vi "TAT_Start.vi"(8 "error In":errorcluster) -> (0 "error out":errorcluster)   [LabVIEW 2017]
uses:
  <vilib>/Utility/error.llb/DialogType.ctl
  Controls/Ass. Loop Control.ctl
  <vilib>/addons/database/Connection.llb/Conn ObjectReference.ctl
  2ffc4e95-467e-4723-8c12-a792954531b5.vi
  <vilib>/addons/database/Connection.llb/DB Tools Open Connec (Path).vi
  Global/Global 1.vi
  <vilib>/Instr/_visa.llb/VISA Configure Serial Port (Instr).vi
  <vilib>/addons/database/NI_Database_API.lvlib
  8539105e-fe5f-4c29-a376-e00596b22cdb.vi
  <vilib>/Utility/config.llb/NI_LVConfig.lvlib
panel:
  out "Para Value":T1
  out "PREVIOUS BARCODE":string
  out "PACKAGED QUANTITY":string
  out "SCANNED QUANTITY":string
  out "PACKAGE STICKER":string
  out "PRN to Print":string
  out "CYCLE RESULT:-":bool caption="LEAK RESULT:-"
  out "CYCLE STATUS STATION 2":string caption="CYCLE STATUS 2:-"
  out "SERIAL NO.:- 2":dbl
  in  "Model Selection:-":string(combo)
  out "CYCLE TIME:-":u32
  out "BARCODE STATION 2":string caption="QR CODE :-"
  out "CYCLE START:-":bool caption="LEAK RESULT:-"
  out "PREVIOUS BARCODE":string[](array[string])
  out "scanned":string
  out "Scanned Qty  2":string
  out "PROJECT :-":string
  out "PACKAGE Qty":string
  out "TORISHI CODE:-":string
  out "PART No.:-":string
  out "PLC STATUS:-":bool
  in  "Stop":bool
  out "QR STATION 1":string caption="QR CODE:-"
  out "RESULT STATION 1":bool caption="FINAL RESULT:-"
  out "USER:-":string
  out "PART NAME :-":string
  in  "ASS-Alarms":bool
  out "CYCLE STATUS STATION 1":string caption="CYCLE STATUS 1:-"
  out "DATE/TIME":string
  # "KAPSE SONS ROBOTICS\n& AUTOMATION"
  # "MODEL SELECTION:-"
  # "MIN"
  # "MAX"
  # "ACTUAL"
  # "STATUS"
  # "BLINKER CURRENT (mA)"
  # "POWER FOLD CURRENT (mA)"
  # "Nm"
  # "GLASS ACTUATOR CURRENT-1 (mA)"
  # "GLASS ACTUATOR CURRENT-2 (mA)"
  # "GROUND (Deg)"
  # "SKY (Deg)"
  # "EXTERIOR (Deg)"
  # "INTERIOR (Deg)"
  # "GLASS PULL OUT LOAD (Kg)"
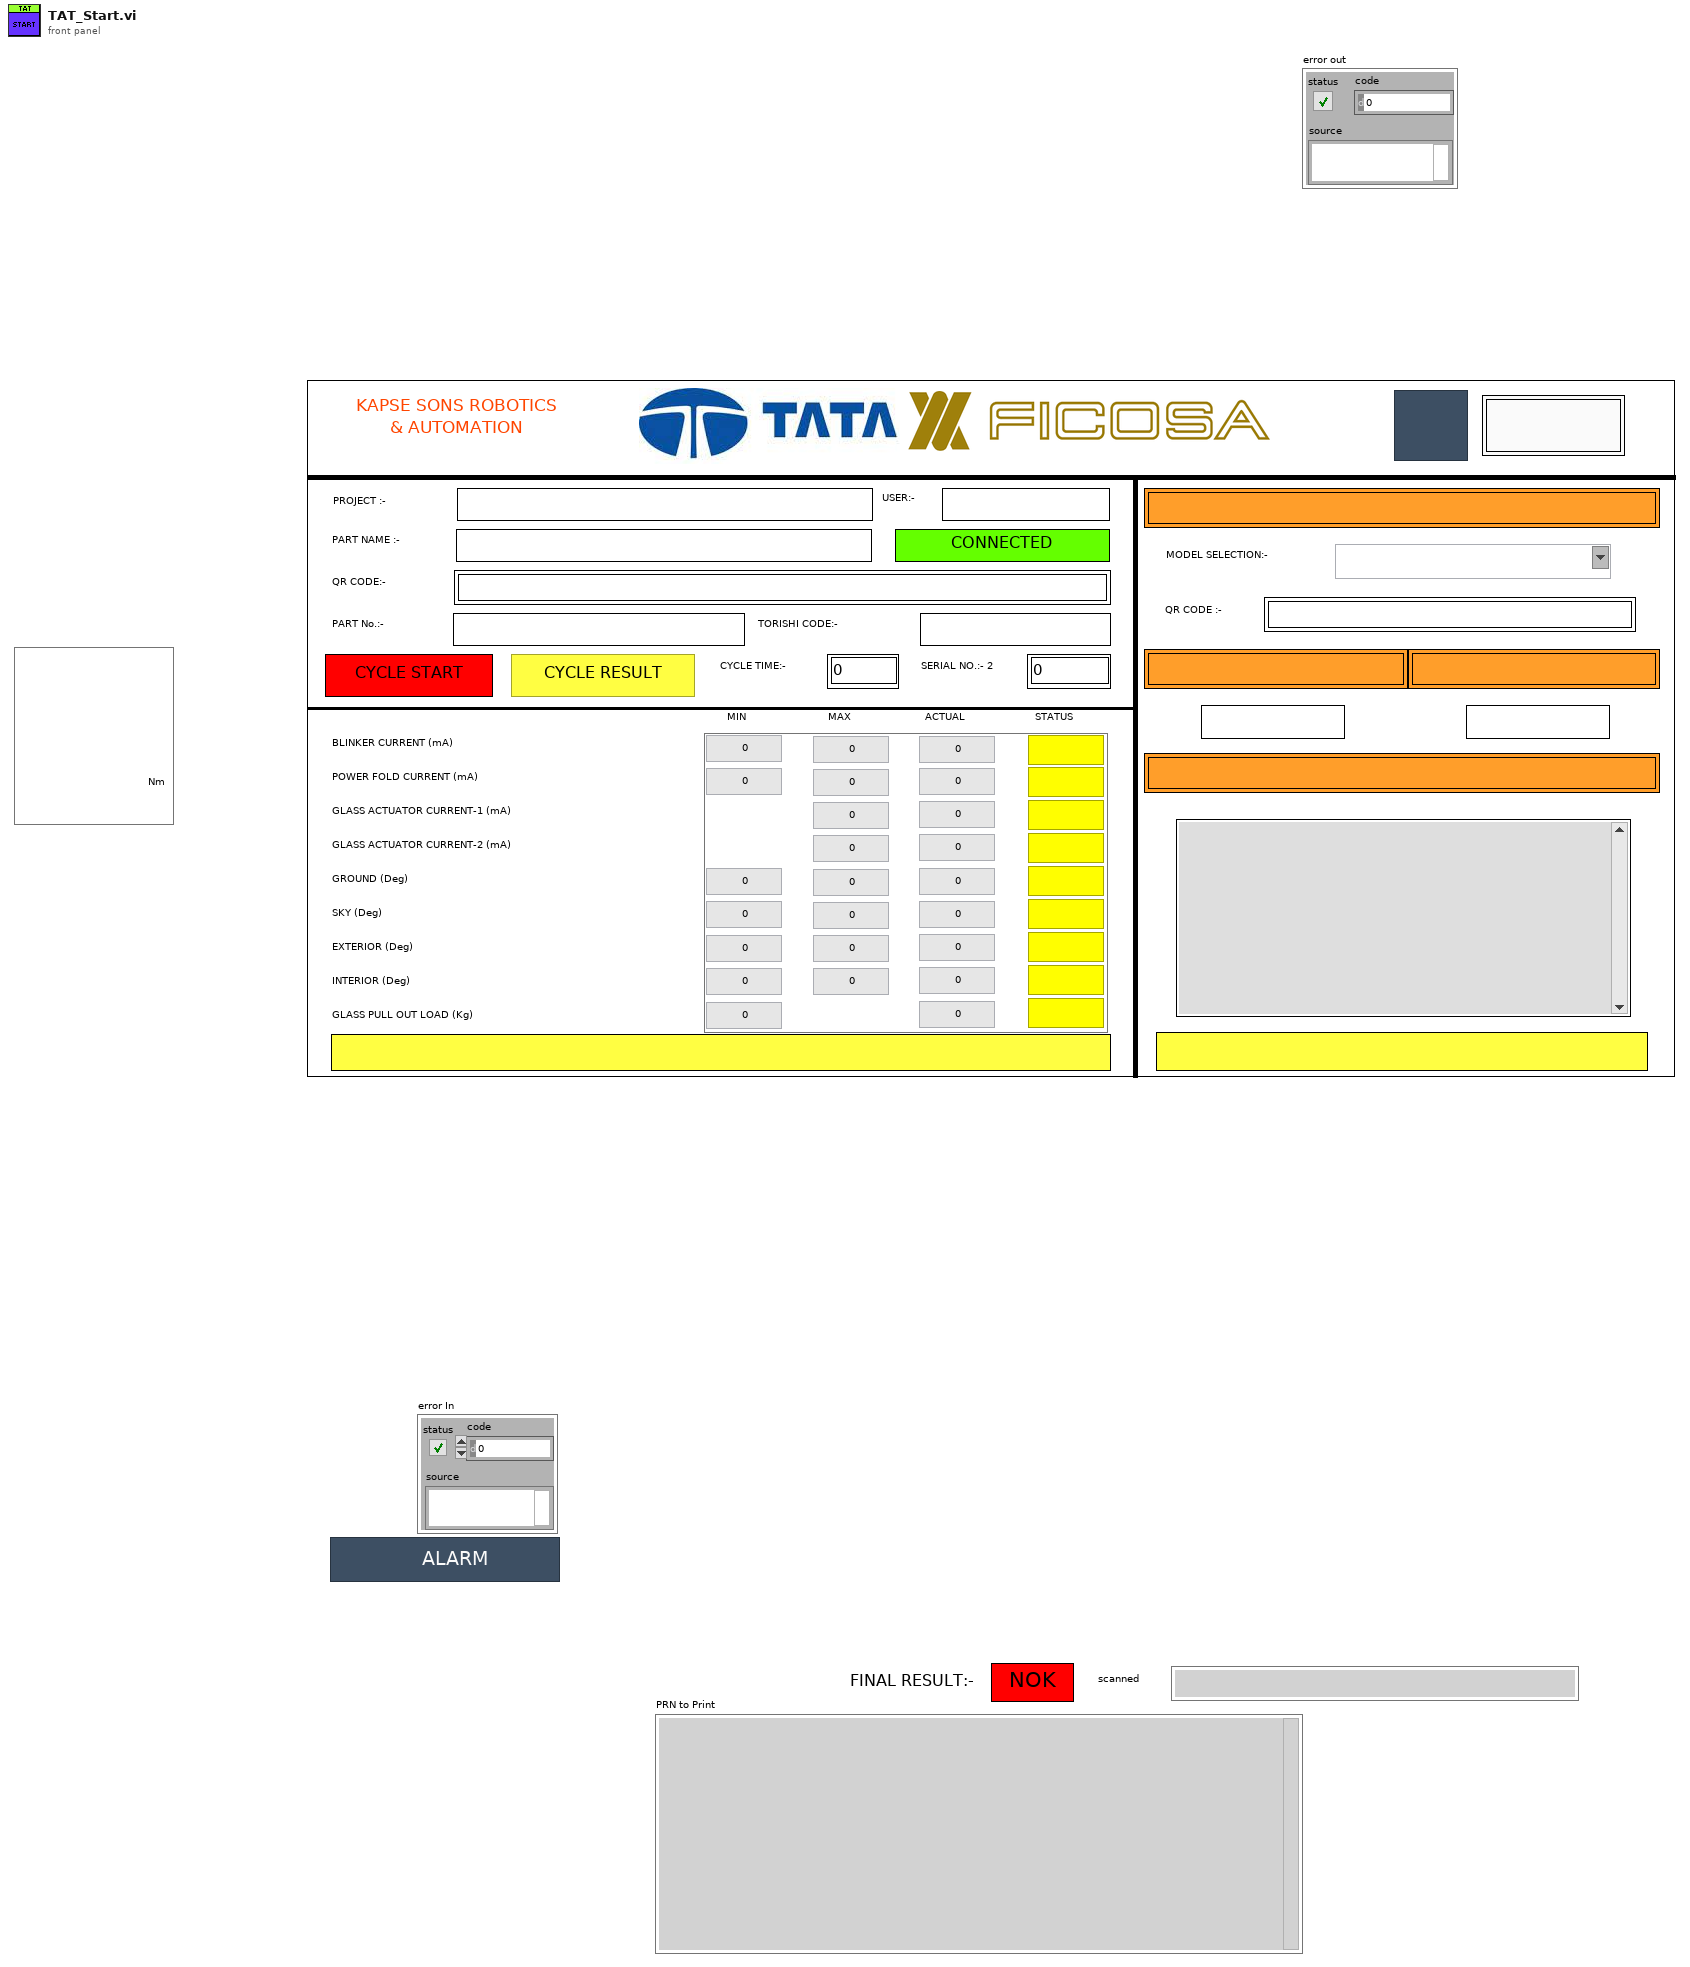
[diagram p1: front panel]
types:
  T1 = cluster{"1.1":dbl, "1.2":dbl, "1.3":dbl, "2.1":dbl, "2.2":dbl, "2.3":dbl, "3.2":dbl, "3.3":dbl, "4.2":dbl, "4.3":dbl, "5.1":dbl, "5.2":dbl, "5.3":dbl, "6.1":dbl, "6.2":dbl, "6.3":dbl, "7.1":dbl, "7.2":dbl, "7.3":dbl, "8.1":dbl, "8.2":dbl, "8.3":dbl, "9.1":dbl, "9.3":dbl, "1.4 CYCLE START":bool, "2.4 CYCLE START":bool, "3.4 CYCLE START":bool, "4.4 CYCLE START":bool, "5.4 CYCLE START":bool, "6.4 CYCLE START":bool, "7.4 CYCLE START":bool, "8.4 CYCLE START":bool, "9.4 CYCLE START":bool}
  T2 = typedef "NI_Database_API.lvlib/Conn ObjectReference.ctl" = refnum<k1>
  T3 = cluster{"Varient number":u16, "Part name":string, "connection reference":T2, "Batch_Size":u16, "PART_NO":string, "TORISHI_CODE":string, "scanner com":refnum<visa-resource-name>, "Part Name List":string[], "Varient path":path, "Current Varient path":path, "Communication path":path, "Package path":path, "Part PRN path":path, "Station2 printer IP":string, "Station1 printer IP":string, "Current Serial Number":string, "Station1_QR":string, "Serial_Number":path, "PRIVIOUS code":string[], "Barcode station 2 to log Dn":string, "Barcode station 2 to log Up":string}
  T4 = cluster{"Varient number":u16, "Part name":string, "Barcode":string, "connection reference":T2, "Batch_Size":u16, "PART_NO":string, "TORISHI_CODE":string, "scanner com":refnum<visa-resource-name>, "Part Name List":string[], "Varient path":path, "Current Varient path":path, "Communication path":path, "Package path":path, "Part PRN path":path, "Station2 printer IP":string, "Station1 printer IP":string, "Current Serial Number":string, "Station1_QR":string, "Serial_Number":path, "PRIVIOUS code":string[], "Barcode station 2 to log":string}
  T5 = typedef "Ass. Loop Control.ctl" = enum16{"Package_Qty_Count", "GENERATE_QR_PRNT", "Cluster_update", "Waiting_for_scan", "barcode CHECK", "Int", "SaveReport ", "Barcode Print", "Start Cycle", "Wait", "Cycle End", "Stop"}
  T6 = typedef "DialogType.ctl" = u16
  T7 = enum32{"invalid app kind", "Development System", "Run Time System", "Student Edition", "Embedded LabVIEW", "Evaluation", "Custom"}
  T8 = typedef "NI_LVConfig.lvlib/Config Data RefNum.ctl" = refnum<k1>
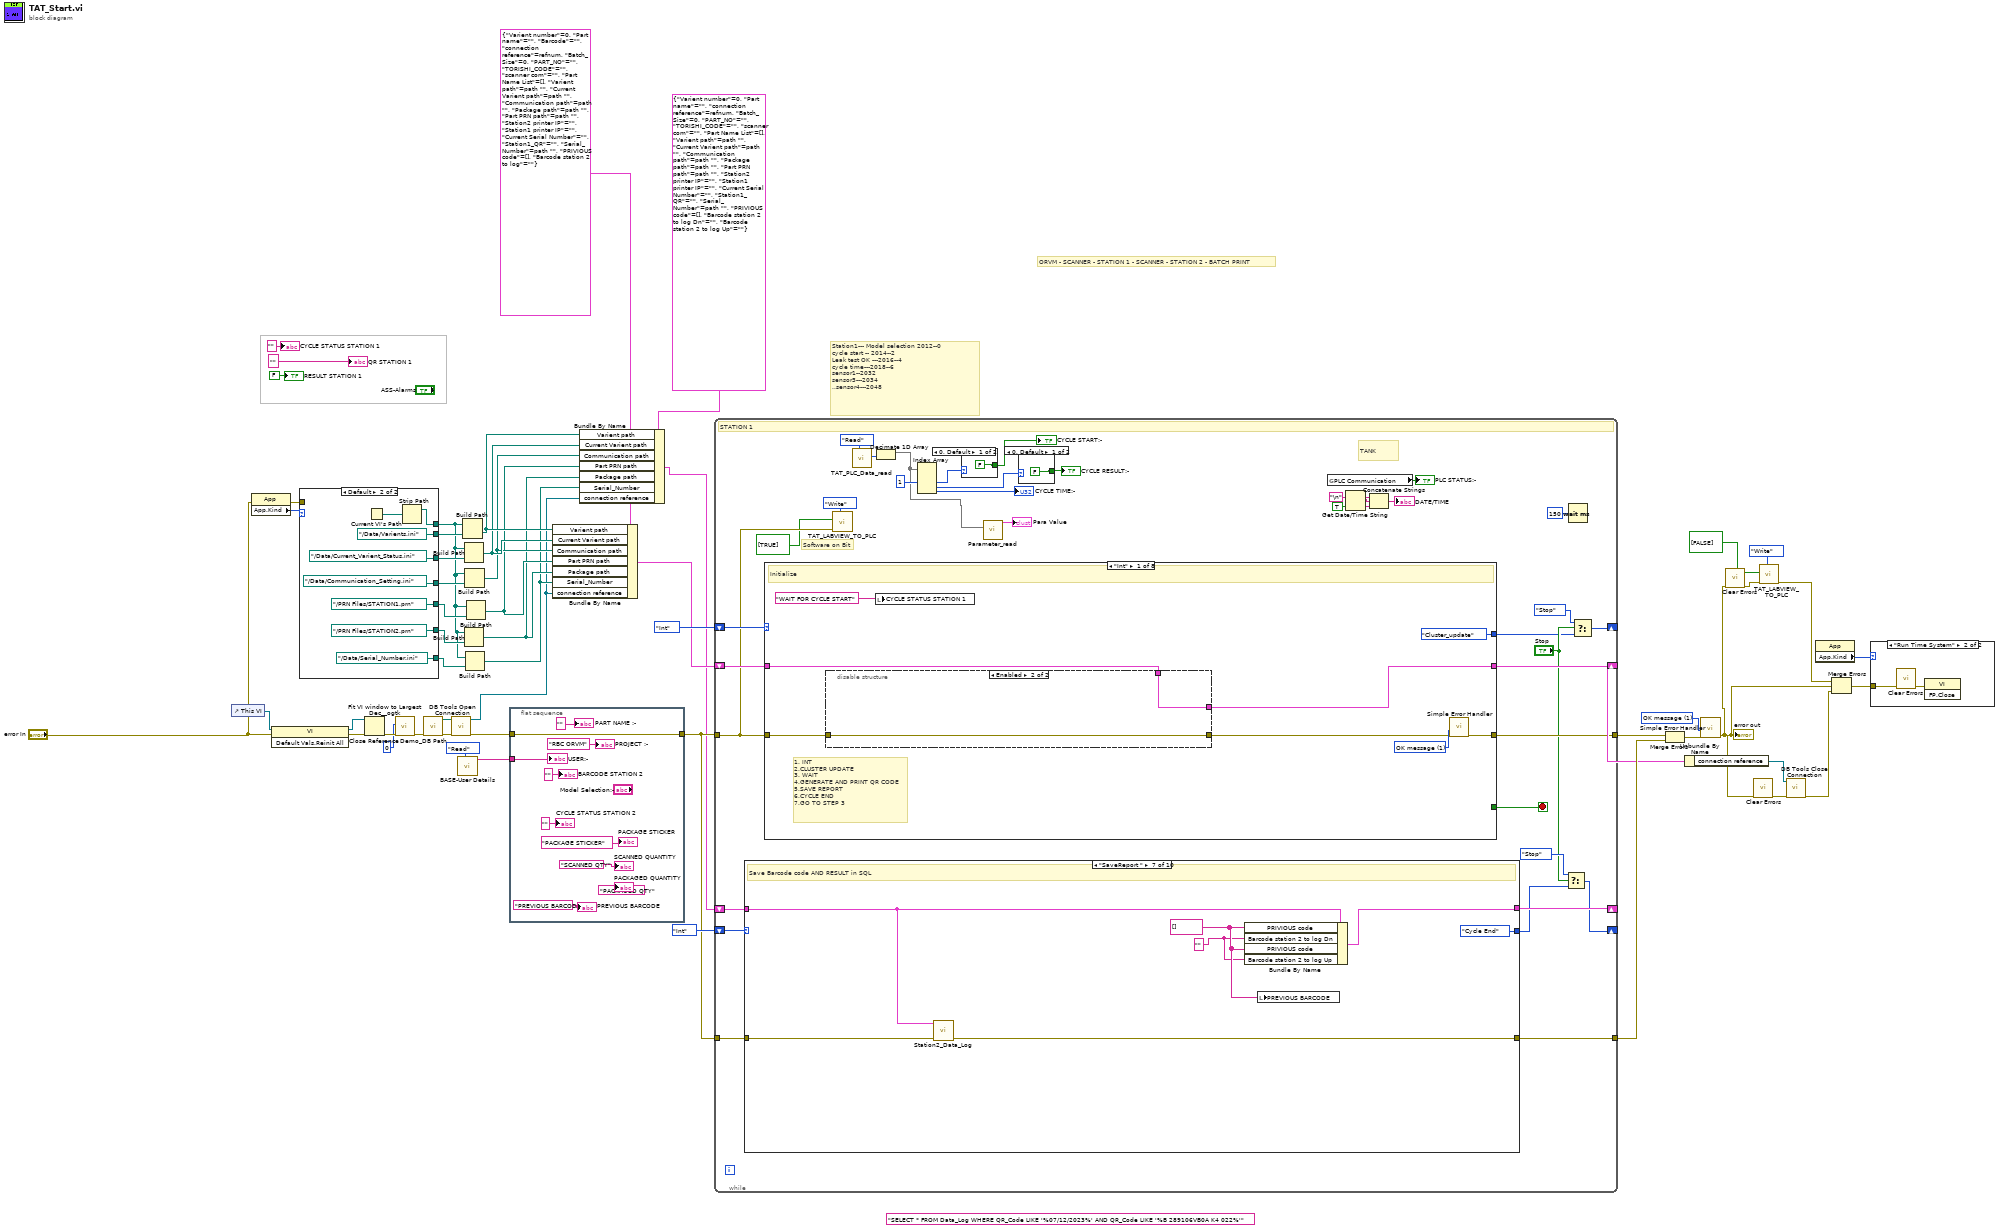
[diagram p0: block diagram]
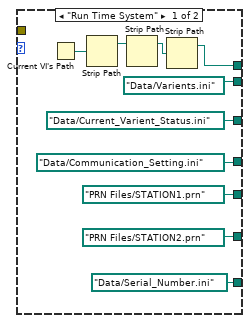
[diagram p2: hidden frame]
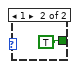
[diagram p4: hidden frame]
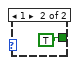
[diagram p5: hidden frame]
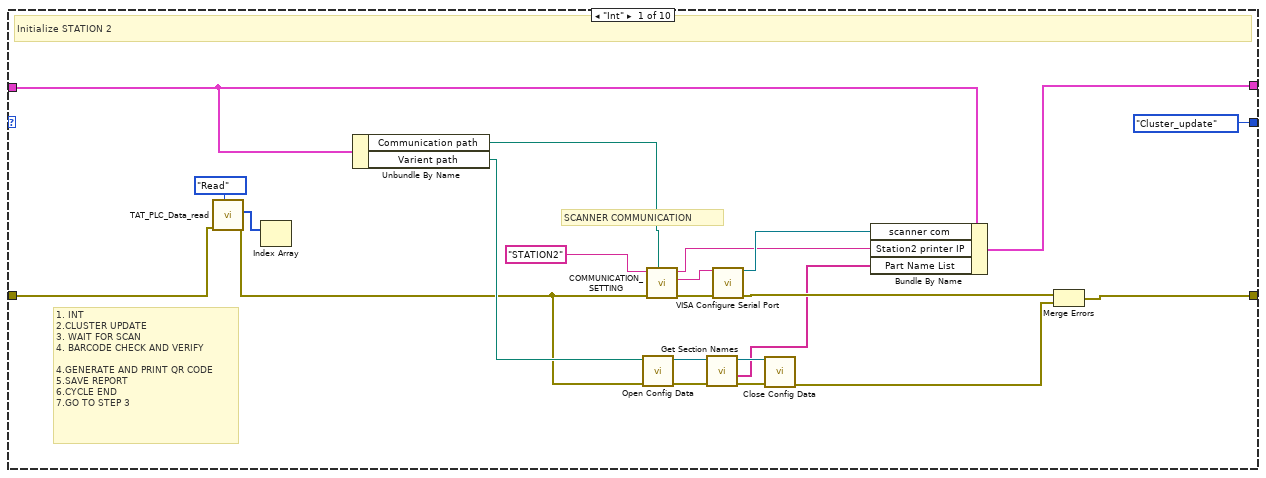
[diagram p6: hidden frame]
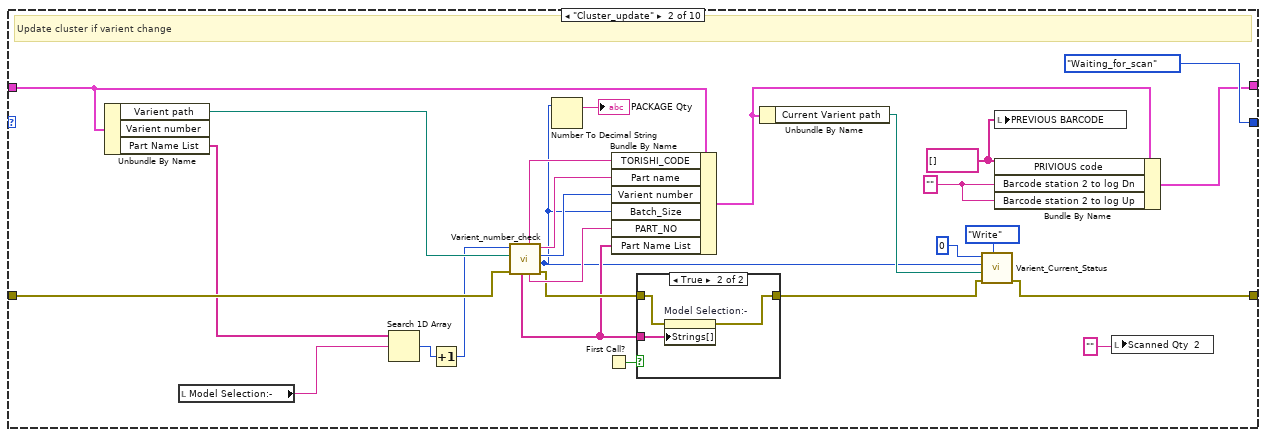
[diagram p7: hidden frame]
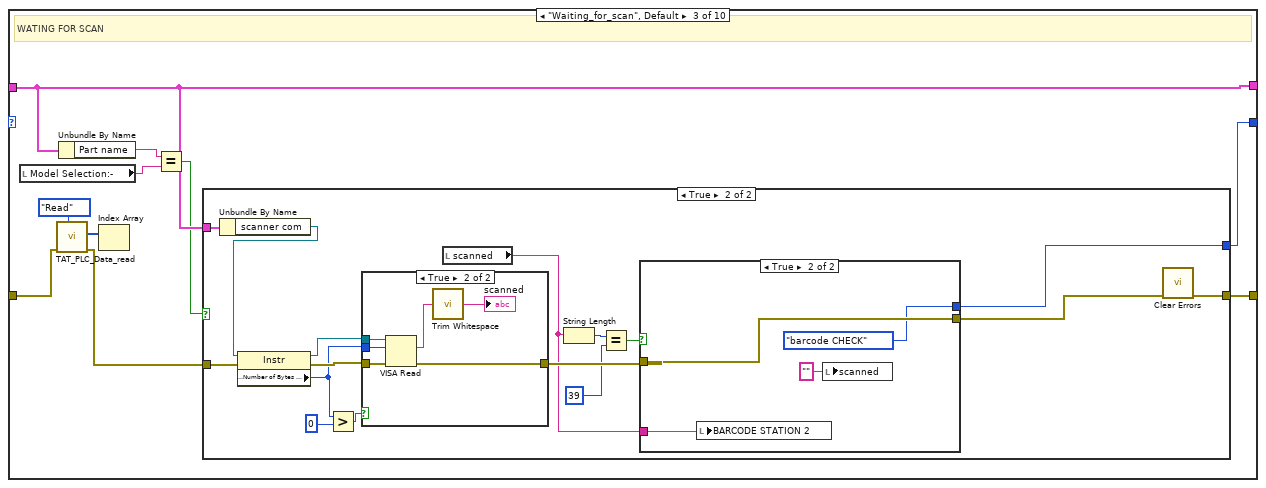
[diagram p9: hidden frame]
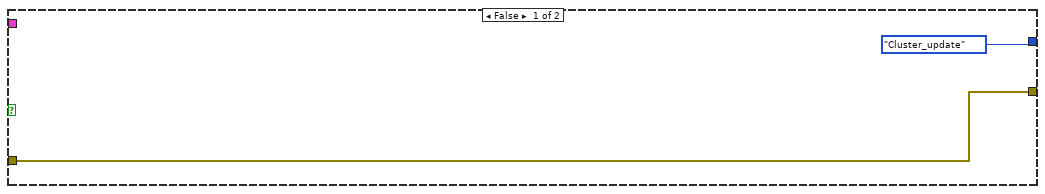
[diagram p10: hidden frame]
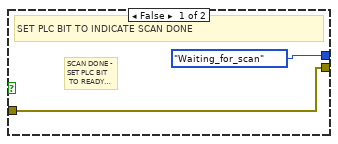
[diagram p12: hidden frame]
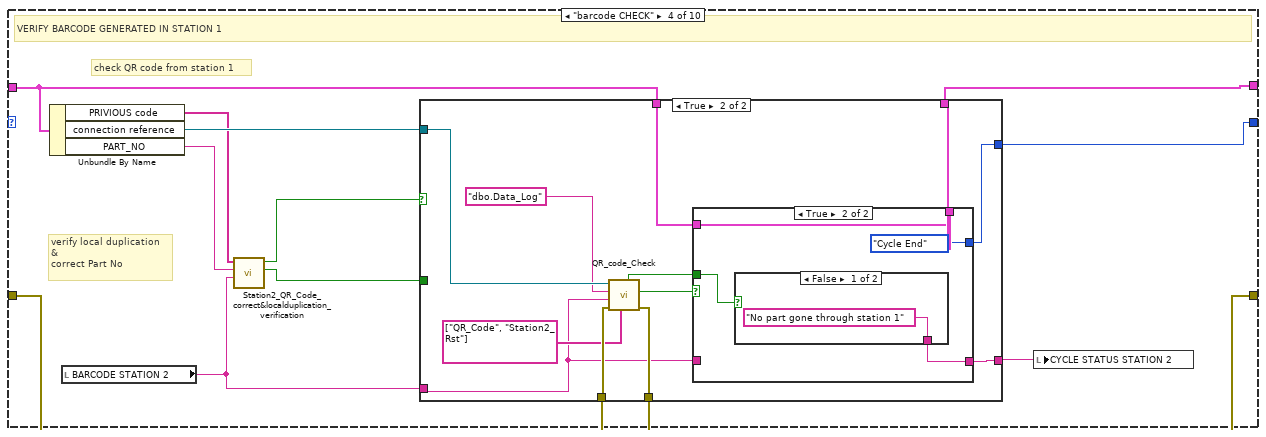
[diagram p13: hidden frame]
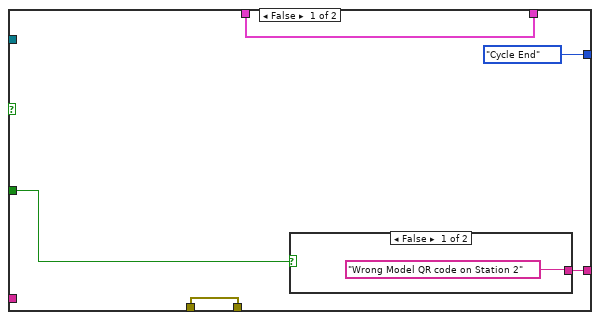
[diagram p14: hidden frame]
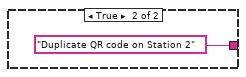
[diagram p15: hidden frame]
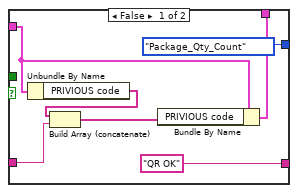
[diagram p16: hidden frame]
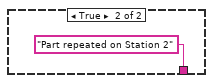
[diagram p17: hidden frame]
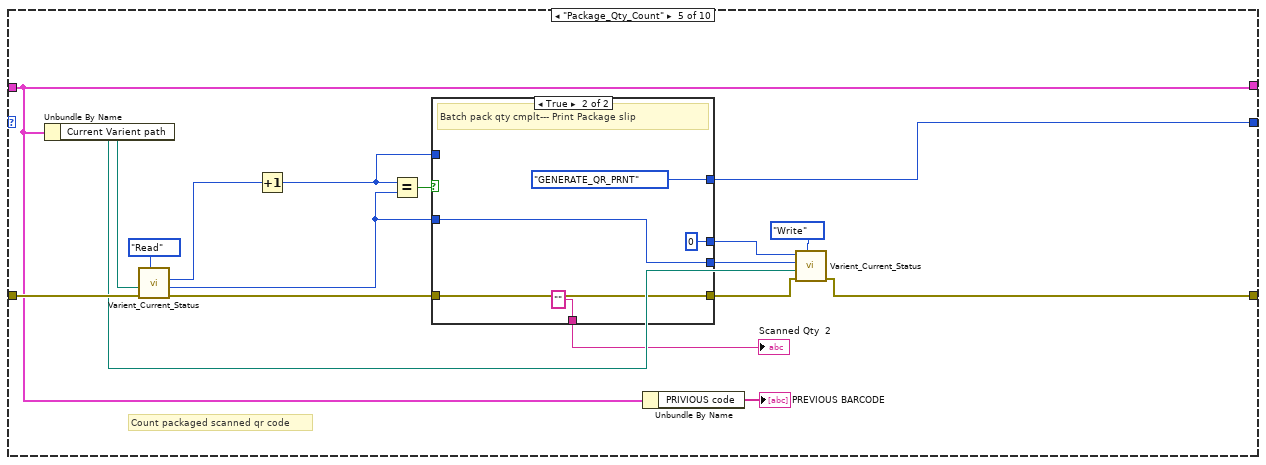
[diagram p18: hidden frame]
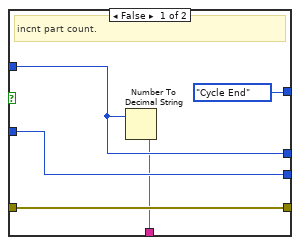
[diagram p19: hidden frame]
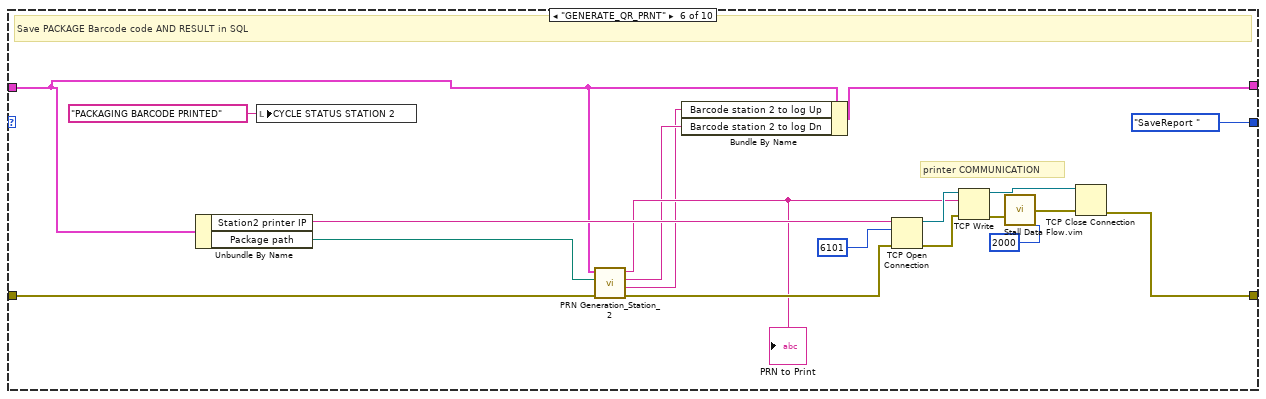
[diagram p20: hidden frame]
diagram:
  (unwired) "SELECT * FROM Data_Log WHERE QR_Code LIKE '%07/12/2023%' AND QR_Code LIKE '%B 289106VB0A K4 022%'" ("format string")
  w41 = T6 1 items=["no dialog", "OK message", "continue or stop message", "OK message + warnings", "continue/stop + warnings"] ("type of dialog (OK msg:1)")
  # "Station1--- Model selection 2012--0\ncycle start -- 2014--2\nLeak test OK ---2016--4\ncycle time---2018--6\nsensor1--2032\nsensor3---2034\n..sensor4---2048"
  # "ORVM - SCANNER - STATION 1 - SCANNER - STATION 2 - BATCH PRINT"
  n1 = control-ref of="This VI"() -> (w53:refnum<vi>)
  n2 = property class="App"(error in="error In") -> (error out=w31:errorcluster, "App.Kind"=w36:T7)  [unwired: 1 in, 1 out]
  n3 = invoke class="VI" method="Default Vals.Reinit All"(reference=w53, error in="error In") -> (reference out=w51:refnum<vi>, error out=w52:errorcluster)  [unwired: 1 in, 1 out]
  n4 = case shown="Default" w36 {
    tunnel: [path "Data/Varients.ini" ("path") path "../Data/Varients.ini" ("path")] -> w35
    tunnel: [w59 w69] -> w26
    tunnel: [path "Data/Current_Varient_Status.ini" ("path") path "../Data/Current_Varient_Status.ini" ("path")] -> w34
    tunnel: [path "Data/Communication_Setting.ini" ("path") path "../Data/Communication_Setting.ini" ("path")] -> w33
    tunnel: [path "PRN Files/STATION2.prn" ("path") path "../PRN Files/STATION2.prn" ("path")] -> w32
    tunnel: w31 -> [_ _]
    tunnel: [path "PRN Files/STATION1.prn" ("path") path "../PRN Files/STATION1.prn" ("path")] -> w29
    tunnel: [path "Data/Serial_Number.ini" ("path") path "../Data/Serial_Number.ini" ("path")] -> w25
    frame "Run Time System" {
      n5 = Current VI's Path() -> (path=w62:path)
      n6 = Strip Path(path=w62) -> (stripped path=w61:path)  [unwired: 1 out]
      n7 = Strip Path(path=w61) -> (stripped path=w60:path)  [unwired: 1 out]
      n8 = Strip Path(path=w60) -> (stripped path=w59:path)  [unwired: 1 out]
    }
    frame Default {
      n9 = Current VI's Path() -> (path=w70:path)
      n10 = Strip Path(path=w70) -> (stripped path=w69:path)  [unwired: 1 out]
    }
  }
  n11 = Close Reference(reference=w51, error in (no error)=w52) -> (error out=w50:errorcluster)
  n12 = call <userlib>:"Fit VI window to Largest Dec__ogtk.vi"("error in (no error)"=w50, "border spacing (2 px)"=0) -> ("error out"=w20:errorcluster)  [unwired: 4 in, 1 out]
  n13 = call "Demo_DB Path.vi"("error in"=w20) -> ("error out"=w22:errorcluster, "DB Path"=w21:path)  [unwired: 9 in]
  n14 = call-poly <vilib>:"DB Tools Open Connection.vi"("error in (no error)"=w22, "connection information"=w21) -> ("error out"=w19:errorcluster, "connection reference"=w9:T2)  [unwired: 6 in]
  n15 = call "BASE-User Details.vi"("Enum"=enum16{"Read", "Write"}."Read") -> ("User Name Out"=w42:string)  [unwired: 9 in, 1 out]
  n16 = Build Path(base path=w26, name or relative path=w35) -> (appended path=w15:path)
  n17 = Build Path(base path=w26, name or relative path=w34) -> (appended path=w14:path)
  n18 = Build Path(base path=w26, name or relative path=w32) -> (appended path=w11:path)
  n19 = Build Path(base path=w26, name or relative path=w33) -> (appended path=w13:path)
  n20 = Build Path(base path=w26, name or relative path=w25) -> (appended path=w10:path)
  n21 = Build Path(base path=w26, name or relative path=w29) -> (appended path=w12:path)
  n22 = flat-sequence {
    tunnel: [w81] -> w39
    tunnel: w19 -> [w81]
    tunnel: w42 -> [w79]
    frame #0 {
      "USER:-" <- w79
      "PART NAME :-" <- ""
      "PROJECT :-" <- "RBC ORVM" ("PROJECT")
      "BARCODE STATION 2" <- "" ("BARCODE STATION 2")
      "CYCLE STATUS STATION 2" <- "" ("CYCLE STATUS STATION 2")
      "PACKAGE STICKER" <- "PACKAGE STICKER" ("PACKAGE STICKER")
      "SCANNED QUANTITY" <- "SCANNED QTY" ("PACKAGE STICKER")
      "PACKAGED QUANTITY" <- "PACKAGED QTY" ("PACKAGE STICKER")
      "PREVIOUS BARCODE" <- "PREVIOUS BARCODE" ("PACKAGE STICKER")
    }
  }
  n23 = Bundle By Name(cluster=T4 {"Varient number"=0, "Part name"="", "Barcode"="", "connection reference"=refnum, "Batch_Size"=0, "PART_NO"="", "TORISHI_CODE"="", "scanner com"="", "Part Name List"=[], "Varient path"=path "", "Current Varient path"=path "", "Communication path"=path "", "Package path"=path "", "Part PRN path"=path "", "Station2 printer IP"="", "Station1 printer IP"="", "Current Serial Number"="", "Station1_QR"="", "Serial_Number"=path "", "PRIVIOUS code"=[], "Barcode station 2 to log"=""}, "Varient path"=w15, "Current Varient path"=w14, "Communication path"=w13, "Part PRN path"=w12, "Package path"=w11, "Serial_Number"=w10, "connection reference"=w9) -> (w27:T4)
  n24 = Bundle By Name(cluster=T3 {"Varient number"=0, "Part name"="", "connection reference"=refnum, "Batch_Size"=0, "PART_NO"="", "TORISHI_CODE"="", "scanner com"="", "Part Name List"=[], "Varient path"=path "", "Current Varient path"=path "", "Communication path"=path "", "Package path"=path "", "Part PRN path"=path "", "Station2 printer IP"="", "Station1 printer IP"="", "Current Serial Number"="", "Station1_QR"="", "Serial_Number"=path "", "PRIVIOUS code"=[], "Barcode station 2 to log Dn"="", "Barcode station 2 to log Up"=""}, "Varient path"=w15, "Current Varient path"=w14, "Communication path"=w13, "Part PRN path"=w12, "Package path"=w11, "Serial_Number"=w10, "connection reference"=w9) -> (w7:T3)
  n25 = while {
    tunnel: w39 -> [w83]
    shift-right: [w113] -> _
    shift-left: Ass._Loop_Control."Int" ("Enum") -> [w118]
    shift-right: [w116] -> w16
    shift-left: w27 -> [w115]
    tunnel: [w114] -> w46
    shift-right: [w99] -> _
    shift-left: Ass._Loop_Control."Int" ("Enum") -> [w105]
    tunnel: w39 -> [w104]
    shift-right: [w102] -> _
    shift-left: w7 -> [w103]
    tunnel: [w101] -> w38
    stop <- w106 stop-if-true
    # "Software on Bit"
    # "TANK"
    # "STATION 1"
    n26 = case shown="\"SaveReport \"" w105 {
      tunnel: [Ass._Loop_Control."Cluster_update" ("Enum") Ass._Loop_Control."Waiting_for_scan" ("Enum") w184 w221 w265 Ass._Loop_Control."SaveReport " ("Enum") Ass._Loop_Control."Cycle End" ("Enum") Ass._Loop_Control."Waiting_for_scan" ("Enum") Ass._Loop_Control."Stop" ("Enum") Ass._Loop_Control."Wait" ("Enum")] -> w98
      tunnel: [w141 w147 w179 w227 w264 w290 w311 w314 w319 w323] -> w102
      tunnel: [w129 w153 w185 w225 w271 w297 w310 w315 w320 w324] -> w101
      tunnel: w104 -> [w124 w170 w181 w226 w277 w295 w312 w315 w317 w324]
      tunnel: w103 -> [w137 w163 w179 w228 w264 w291 w309 w314 w319 w323]
      frame "Int" {
        # "1. INT\n2.CLUSTER UPDATE\n3. WAIT FOR SCAN\n4. BARCODE CHECK AND VERIFY\n\n4.GENERATE AND PRINT QR CODE\n5.SAVE REPORT\n6.CYCLE END\n7.GO TO STEP 3"
        # "SCANNER COMMUNICATION"
        # "Initialize STATION 2"
        n27 = call "TAT_PLC_Data_read.vi"("Enum"=enum16{"Read", "Write"}."Read", "error in (no error)"=w124) -> ("error out"=w123:errorcluster, "Array 2"=w126:u16[])  [unwired: 8 in]
        n28 = Index Array(array=w126) -> ()  [unwired: 1 in, 1 out]
        n29 = Unbundle By Name(w137) -> ("Communication path"=w136:path, "Varient path"=w127:path)
        n30 = call <vilib>:"Open Config Data.vi"("error in (no error)"=w123, "configuration file path"=w127) -> ("error out"=w134:errorcluster, "refnum"=w135:T8)  [unwired: 7 in, 1 out]
        n31 = call "COMMUNICATION_SETTING.vi"("communication path"=w136, "error in"=w123, "STATION"="STATION2") -> ("error out"=w143:errorcluster, "SCAN_COM"=w139:string, "PRINT_COM"=w138:string)  [unwired: 6 in]
        n32 = call <vilib>:"Get Section Names.vi"("error in (no error)"=w134, "refnum"=w135) -> ("error out"=w133:errorcluster, "section names"=w128:string[], "refnum out"=w132:T8)  [unwired: 7 in]
        n33 = call-poly "VISA Configure Serial Port"("VISA resource name"=w139, "error in (no error)"=w143) -> ("VISA resource name out"=w140:refnum<visa-resource-name>, "error out"=w130:errorcluster)  [unwired: 12 in]
        n34 = call <vilib>:"Close Config Data.vi"("error in (no error)"=w133, "refnum"=w132) -> ("error out"=w131:errorcluster)  [unwired: 8 in, 1 out]
        n35 = Bundle By Name(cluster=w137, "scanner com"=w140, "Station2 printer IP"=w138, "Part Name List"=w128) -> (w141:T3)
        n36 = Merge Errors(w130, w131) -> (w129:errorcluster)
      }
      frame "Cluster_update" {
        w145 = "" ("Barcode station 2 to log")
        w146 = string[] [] ("PREVIOUS Code")
        # "Update cluster if varient change"
        n37 = Unbundle By Name(w163) -> ("Varient path"=w169:path, "Part Name List"=w160:string[])  [unwired: 1 out]
        n38 = local read "Model Selection:-"() -> (w158:string)
        n39 = Search 1D Array(1D array=w160, element=w158) -> (index of element=w162:i32)  [unwired: 1 in]
        n40 = Increment(x=w162) -> (x+1=w159:i32)
        n41 = call "Varient_number_check.vi"("error in"=w170, "Varient path"=w169, "Varient No."=w159) -> ("error out"=w164:errorcluster, "Batch Size"=w151:i32, "Varient Number"=w156:i32, "Part Name"=w167:string, "PART_NO"=w166:string, "TORISHI_CODE"=w168:string, "MODEL LIST"=w161:string[])  [unwired: 2 in]
        n42 = Number To Decimal String(number=w151) -> (decimal integer string=→"PACKAGE Qty":string)  [unwired: 1 in]
        n43 = First Call?() -> (First Call?: T/F=w157:bool)
        n44 = Bundle By Name(cluster=w163, "TORISHI_CODE"=w168, "Part name"=w167, "Varient number"=w156, "Batch_Size"=w151, "PART_NO"=w166, "Part Name List"=w161) -> (w148:T3)
        n45 = case shown="True" w157 {
          tunnel: w164 -> [w172 w175]
          tunnel: [w172 w174] -> w154
          tunnel: w161 -> [_ w173]
          frame False {
          }
          frame True {
            n46 = property on="Model Selection:-" class="CmbBox"(error in=w175, "Strings[]"=w173) -> (error out=w174:errorcluster)  [unwired: 1 in, 1 out]
          }
        }
        n47 = Unbundle By Name(w148) -> ("Current Varient path"=w152:path)
        n48 = call "Varient_Current_Status.vi"("Enum"=enum16{"Write", "Read"}."Write", "error in"=w154, "Current Varient Status"=w152, "Batch Size"=w151, "Varient count"=0) -> ("error out"=w153:errorcluster)  [unwired: 4 in, 2 out]
        n49 = local write "PREVIOUS BARCODE"(w146) -> ()
        n50 = Bundle By Name(cluster=w148, "PRIVIOUS code"=w146, "Barcode station 2 to log Dn"=w145, "Barcode station 2 to log Up"=w145) -> (w147:T3)
        n51 = local write "Scanned Qty  2"("") -> ()
      }
      frame "Waiting_for_scan", Default {
        # "WATING FOR SCAN"
        n52 = local read "Model Selection:-"() -> (w177:string)
        n53 = call "TAT_PLC_Data_read.vi"("Enum"=enum16{"Read", "Write"}."Read", "error in (no error)"=w181) -> ("error out"=w180:errorcluster, "Array 2"=w183:u16[])  [unwired: 8 in]
        n54 = Unbundle By Name(w179) -> ("Part name"=w178:string)
        n55 = Index Array(array=w183) -> ()  [unwired: 1 in, 1 out]
        n56 = Equal?(x=w178, y=w177) -> (x = y?=w176:bool)
        n57 = case shown="True" w176 {
          tunnel: [w187 w203] -> w185
          tunnel: [Ass._Loop_Control."Cluster_update" ("Enum") w198] -> w184
          tunnel: w180 -> [w187 w197]
          tunnel: w179 -> [_ w196]
          frame False {
          }
          frame True {
            n58 = Unbundle By Name(w196) -> ("scanner com"=w195:refnum<visa-resource-name>)
            n59 = property class="Instr"(reference=w195, error in=w197) -> (reference out=w202:refnum<visa-resource-name>, error out=w201:errorcluster, "Serial Settings:Number of Bytes at Serial Port"=w188:u32)
            n60 = Greater?(x=w188, y=u32 0) -> (0:w189:bool)
            n61 = case shown="True" w189 {
              tunnel: w202 -> [_ w210]
              tunnel: w201 -> [w204 w209]
              tunnel: w188 -> [_ w208]
              tunnel: [w204 w207] -> w200
              frame False {
              }
              frame True {
                n62 = VISA Read(VISA resource name=w210, byte count=w208, error in (no error)=w209) -> (read buffer=w206:string, error out=w207:errorcluster)  [unwired: 2 out]
                n63 = call <vilib>:"Trim Whitespace.vi"("string"=w206) -> ("trimmed string"=→"scanned":string)  [unwired: 1 in]
              }
            }
            n64 = local read "scanned"() -> (w192:string)
            n65 = String Length(string=w192) -> (length=w194:i32)
            n66 = Equal?(x=w194, y=39) -> (x = y?=w191:bool)
            n67 = case shown="True" w191 {
              tunnel: w200 -> [w212 w216]
              tunnel: [w212 w216] -> w199
              tunnel: w192 -> [_ w213]
              tunnel: [Ass._Loop_Control."Waiting_for_scan" ("Enum") Ass._Loop_Control."barcode CHECK" ("Enum")] -> w198
              frame False {
                # "SCAN DONE - SET PLC BIT\n TO READY CYCLE"
                # "SET PLC BIT TO INDICATE SCAN DONE"
              }
              frame True {
                n68 = local write "BARCODE STATION 2"(w213) -> ()
                n69 = local write "scanned"("" ("scanned")) -> ()
              }
            }
            n70 = call <vilib>:"Clear Errors.vi"("error in (no error)"=w199) -> ("error out"=w203:errorcluster)  [unwired: 5 in, 1 out]
          }
        }
      }
      frame "barcode CHECK" {
        # "verify local duplication\n&\ncorrect Part No"
        # "check QR code from station 1"
        # "VERIFY BARCODE GENERATED IN STATION 1"
        n71 = Unbundle By Name(w228) -> ("PRIVIOUS code"=w220:string[], "connection reference"=w224:T2, "PART_NO"=w223:string)
        n72 = local read "BARCODE STATION 2"() -> (w219:string)
        n73 = call "Station2_QR_Code_correct&localduplication_verification.vi"("BARCODE STATION in"=w219, "PART_NO"=w223, "PRIVIOUS code"=w220) -> ("Correct part no True"=w217:bool, "Correct part no & No duplication TRUE"=w218:bool)  [unwired: 7 in]
        n74 = case shown="True" w218 {
          tunnel: w228 -> [w233 w247]
          tunnel: [w233 w246] -> w227
          tunnel: w226 -> [w232 w245]
          tunnel: [w232 w244] -> w225
          tunnel: w224 -> [_ w243]
          tunnel: w219 -> [_ w238]
          tunnel: [w231 w240] -> w222
          tunnel: [Ass._Loop_Control."Cycle End" ("Enum") w239] -> w221
          tunnel: w217 -> [w229 _]
          frame False {
            n75 = case shown="False" w229 {
              tunnel: ["Wrong Model QR code on Station 2" ("Cycle Status") "Duplicate QR code on Station 2" ("Cycle Status")] -> w231
              frame False {
              }
              frame True {
              }
            }
          }
          frame True {
            n76 = call "QR_code_Check.vi"("Columns"=string[] ["QR_Code", "Station2_Rst"] ("columns 2"), "error in (no error)"=w245, "replace %s"=w238, "table"="dbo.Data_Log", "Refnum in"=w243) -> ("error out"=w244:errorcluster, "FALSE healty"=w237:bool, "TRUE Duplication on Station 2"=w236:bool)  [unwired: 1 in, 2 out]
            n77 = case shown="True" w237 {
              tunnel: ["QR OK" ("Cycle Status") w258] -> w240
              tunnel: w247 -> [w251 w257]
              tunnel: [w253 w257] -> w246
              tunnel: [Ass._Loop_Control."Package_Qty_Count" ("Enum") Ass._Loop_Control."Cycle End" ("Enum")] -> w239
              tunnel: w238 -> [w248 _]
              tunnel: w236 -> [_ w255]
              frame False {
                n78 = Unbundle By Name(w251) -> ("PRIVIOUS code"=w250:string[])
                n79 = Build Array (concatenate)(w250, w248) -> (w249:string[])
                n80 = Bundle By Name(cluster=w251, "PRIVIOUS code"=w249) -> (w253:T3)
              }
              frame True {
                n81 = case shown="False" w255 {
                  tunnel: ["No part gone through station 1" ("Cycle Status") "Part repeated on Station 2" ("Cycle Status")] -> w258
                  frame False {
                  }
                  frame True {
                  }
                }
              }
            }
          }
        }
        n82 = local write "CYCLE STATUS STATION 2"(w222) -> ()
      }
      frame "Package_Qty_Count" {
        # "Count packaged scanned qr code"
        n83 = Unbundle By Name(w264) -> ("Current Varient path"=w263:path)
        n84 = call "Varient_Current_Status.vi"("Enum"=enum16{"Write", "Read"}."Read", "error in"=w277, "Current Varient Status"=w263) -> ("error out"=w275:errorcluster, "Batch Size"=w268:i32, "Varient Count"=w274:i32)  [unwired: 6 in]
        n85 = Increment(x=w274) -> (x+1=w269:i32)
        n86 = Equal?(x=w269, y=w268) -> (x = y?=w273:bool)
        n87 = case shown="True" w273 {
          tunnel: [w282 w287] -> w270
          tunnel: w275 -> [w282 w287]
          tunnel: w269 -> [w279 _]
          tunnel: w268 -> [w281 w286]
          tunnel: [w281 w286] -> w267
          tunnel: [w279 0] -> w266
          tunnel: [Ass._Loop_Control."Cycle End" ("Enum") Ass._Loop_Control."GENERATE_QR_PRNT" ("Enum")] -> w265
          tunnel: [w278 "" ("String")] -> w262
          frame False {
            # "incnt part count."
            n88 = Number To Decimal String(number=w279) -> (decimal integer string=w278:string)  [unwired: 1 in]
          }
          frame True {
            # "Batch pack qty cmplt--- Print Package slip"
          }
        }
        "Scanned Qty  2" <- w262
        n89 = Unbundle By Name(w264) -> ("PRIVIOUS code"=→"PREVIOUS BARCODE":string[])
        n90 = call "Varient_Current_Status.vi"("Enum"=enum16{"Write", "Read"}."Write", "error in"=w270, "Current Varient Status"=w263, "Batch Size"=w267, "Varient count"=w266) -> ("error out"=w271:errorcluster)  [unwired: 4 in, 2 out]
      }
      frame "GENERATE_QR_PRNT" {
        # "printer COMMUNICATION"
        # "Save PACKAGE Barcode code AND RESULT in SQL"
        n91 = Unbundle By Name(w291) -> ("Station2 printer IP"=w296:string, "Package path"=w293:path)
        n92 = local write "CYCLE STATUS STATION 2"("PACKAGING BARCODE PRINTED" ("Cycle Status")) -> ()
        n93 = call "PRN Generation_Station_2.vi"("error in (no error)"=w295, "PRN path"=w293, "Cluster"=w291) -> ("error out"=w294:errorcluster, "Barcode Station 2 Up"=w288:string, "Barcode station 2 Dn"=w289:string, "PRN to Print"=w292:string)  [unwired: 5 in]
        "PRN to Print" <- w292
        n94 = Bundle By Name(cluster=w291, "Barcode station 2 to log Up"=w288, "Barcode station 2 to log Dn"=w289) -> (w290:T3)
        n95 = TCP Open Connection(address=w296, remote port or service name=u16 6101, error in (no error)=w294) -> (connection ID=w302:refnum<k5>, error out=w303:errorcluster)  [unwired: 2 in]
        n96 = TCP Write(connection ID=w302, data in=w292, error in (no error)=w303) -> (connection ID out=w300:refnum<k5>, error out=w304:errorcluster)  [unwired: 1 in, 1 out]
        n97 = call "Stall Data Flow.vim"("value in"=w304, "milliseconds to wait"=u32 2000) -> ("value out"=w301:errorcluster)  [unwired: 1 out]
        n98 = TCP Close Connection(connection ID=w300, error in (no error)=w301) -> (error out=w297:errorcluster)  [unwired: 1 in, 1 out]
      }
      frame "SaveReport " {
        w307 = "" ("Barcode station 2 to log")
        w308 = string[] [] ("PREVIOUS Code")
        # "Save Barcode code AND RESULT in SQL"
        n99 = call "Station2_Data_Log.vi"("error in (no error)"=w312, "Cluster"=w309) -> ("error out"=w310:errorcluster)  [unwired: 9 in]
        n100 = Bundle By Name(cluster=w309, "PRIVIOUS code"=w308, "Barcode station 2 to log Dn"=w307, "PRIVIOUS code"=w308, "Barcode station 2 to log Up"=w307) -> (w311:T3)
        n101 = local write "PREVIOUS BARCODE"(w308) -> ()
      }
      frame "Cycle End" {
      }
      frame "Stop" {
        n102 = local write "CYCLE STATUS STATION 2"("STATION STOP" ("Cycle Status")) -> ()
        n103 = Unbundle By Name(w319) -> ("scanner com"=w318:refnum<visa-resource-name>)
        n104 = VISA Close(VISA resource name=w318, error in (no error)=w317) -> (error out=w320:errorcluster)
      }
      frame "Start Cycle" {
        n105 = local write "CYCLE STATUS STATION 1"("Cycle started" ("Cycle Status")) -> ()
      }
    }
    n106 = case shown="\"Int\"" w118 {
      tunnel: [Ass._Loop_Control."Cluster_update" ("Enum") Ass._Loop_Control."Wait" ("Enum") w373 Ass._Loop_Control."Wait" ("Enum") w398 Ass._Loop_Control."Cycle End" ("Enum") Ass._Loop_Control."Wait" ("Enum") Ass._Loop_Control."Stop" ("Enum")] -> w96
      tunnel: [w332 w348 w375 w391 w396 w451 w467 w470] -> w116
      tunnel: w115 -> [w328 w347 w375 w391 w397 w451 w467 w470]
      tunnel: [_ _ FALSE _ _ _ _ TRUE] -> w106
      tunnel: [w330 w350 w362 w388 w392 w445 w466 w468] -> w114
      tunnel: w83 -> [w327 w354 w368 w388 w401 w453 w466 w468]
      frame "Int" {
        w331 = T6 1 items=["no dialog", "OK message", "continue or stop message", "OK message + warnings", "continue/stop + warnings"] ("type of dialog (OK msg:1)")
        # "1. INT\n2.CLUSTER UPDATE\n3. WAIT\n4.GENERATE AND PRINT QR CODE\n5.SAVE REPORT\n6.CYCLE END\n7.GO TO STEP 3"
        # "Initialize"
        n107 = disable-structure shown="Enabled" {
          disable-tunnel: [w340 w342] -> w332
          disable-tunnel: [w339 w343] -> w329
          disable-tunnel: w328 -> [w336 w342]
          disable-tunnel: w327 -> [w335 w343]
          frame Disabled {
            # "printer one removed"
            n108 = Unbundle By Name(w336) -> ("Communication path"=w338:path)
            n109 = call "COMMUNICATION_SETTING.vi"("communication path"=w338, "error in"=w335, "STATION"="STATION1") -> ("error out"=w339:errorcluster, "PRINT_COM"=w337:string)  [unwired: 6 in, 1 out]
            n110 = Bundle By Name(cluster=w336, "Station1 printer IP"=w337) -> (w340:T4)
          }
          frame Enabled {
          }
        }
        n111 = local write "CYCLE STATUS STATION 1"("WAIT FOR CYCLE START" ("Cycle Status")) -> ()
        n112 = call <vilib>:"Simple Error Handler.vi"("type of dialog (OK msg:1)"=w331, "error in (no error)"=w329) -> ("error out"=w330:errorcluster)  [unwired: 3 in, 4 out]
      }
      frame "Cluster_update" {
        # "PART NAME\nPART No.\nPACKAGE QUANTITY\nTORISHI CODE"
        # "PART NAME---\nVARIENT NAME"
        # "Update cluster if varient change"
        n113 = Unbundle By Name(w347) -> ("Varient path"=w346:path)
        n114 = call "TAT_PLC_Data_read.vi"("Enum"=enum16{"Read", "Write"}."Read", "error in (no error)"=w354) -> ("error out"=w351:errorcluster, "Array 2"=w356:u16[])  [unwired: 8 in]
        n115 = Index Array(array=w356) -> (element=w345:u16)  [unwired: 1 in]
        n116 = call "Varient_number_check.vi"("error in"=w351, "Varient path"=w346, "Varient No."=w345) -> ("error out"=w350:errorcluster, "Batch Size"=w349:i32, "Part Name"=w353:string, "PART_NO"=w352:string, "TORISHI_CODE"=w344:string)  [unwired: 2 in, 2 out]
        "PART No.:-" <- w352
        "TORISHI CODE:-" <- w344
        n117 = Bundle By Name(cluster=w347, "Part name"=w353, "Varient number"=w345, "Batch_Size"=w349, "PART_NO"=w352, "TORISHI_CODE"=w344) -> (w348:T4)
        n118 = local write "PART NAME :-"(w353) -> ()
      }
      frame "Wait", Default {
        w364 = T6 1 items=["no dialog", "OK message", "continue or stop message", "OK message + warnings", "continue/stop + warnings"] ("type of dialog (OK msg:1)")
        # "Serial logic"
        # "WAITING FORM CCYLE TO COMPLE TO PRINT QR"
        # "Wait"
        n119 = Unbundle By Name(w375) -> ("Varient number"=w374:u16, "Serial_Number"=w367:path)
        n120 = call "TAT_PLC_Data_read.vi"("Enum"=enum16{"Read", "Write"}."Read", "error in (no error)"=w368) -> ("error out"=w365:errorcluster, "Array 2"=w376:u16[])  [unwired: 8 in]
        n121 = Index Array(array=w376) -> (element #1=w378:u16, element #3=w371:u16, element #5=w360:u16)  [unwired: 5 in, 2 out]
        n122 = Not Equal?(x=w374, y=w378) -> (x != y?=w372:bool)
        n123 = call "Serial_Logic.vi"("error in"=w368, "Serial path"=w367) -> ("error out"=w366:errorcluster)  [unwired: 9 in]
        n124 = Equal?(x=w371, y=u16 1) -> (x = y?=w369:bool)
        n125 = Equal?(x=w360, y=u16 1) -> (x = y?=w359:bool)
        n126 = call <userlib>:"Boolean Trigger__ogtk.vi"("Boolean Input"=w359) -> ("Rising Edge"=w358:bool)  [unwired: 1 in, 1 out]
        n127 = Merge Errors(w365, w366) -> (w363:errorcluster)
        n128 = call <userlib>:"Boolean Trigger__ogtk.vi"("Boolean Input"=w369) -> ("Rising Edge"=w382:bool)  [unwired: 1 in, 1 out]
        n129 = Build Array(w382, w358, w372) -> (w381:bool[])
        n130 = Search 1D Array(1D array=w381, element=TRUE ("Boolean Input")) -> (index of element=w380:i32)  [unwired: 1 in]
        n131 = case shown="1" w380 {
          tunnel: [Ass._Loop_Control."Wait" ("Enum") Ass._Loop_Control."Start Cycle" ("Enum") Ass._Loop_Control."GENERATE_QR_PRNT" ("Enum") Ass._Loop_Control."Cluster_update" ("Enum")] -> w373
          frame -1, Default {
          }
          frame 0 {
            # "CYCYLE START BIT"
          }
          frame 1 {
            # "CYCLE END STORE RLT"
          }
          frame 2 {
            # "CLUSTER UPDATE"
          }
        }
        n132 = call <vilib>:"Simple Error Handler.vi"("type of dialog (OK msg:1)"=w364, "error in (no error)"=w363) -> ("error out"=w362:errorcluster)  [unwired: 3 in, 4 out]
      }
      frame "Start Cycle" {
        n133 = local write "CYCLE STATUS STATION 1"("Cycle started" ("Cycle Status")) -> ()
      }
      frame "GENERATE_QR_PRNT" {
        w394 = T6 1 items=["no dialog", "OK message", "continue or stop message", "OK message + warnings", "continue/stop + warnings"] ("type of dialog (OK msg:1)")
        # "VARIENT NAME REMAIN TO ADD"
        # "GENERATE QR CODE AND PRINT QR CODE"
        n134 = call "TAT_PLC_Data_read.vi"("Enum"=enum16{"Read", "Write"}."Read", "error in (no error)"=w401) -> ("error out"=w400:errorcluster, "Array 2"=w402:u16[])  [unwired: 8 in]
        n135 = Index Array(array=w402) -> (element #5=w395:u16)  [unwired: 5 in, 4 out]
        n136 = case shown="1" w395 {
          tunnel: w400 -> [w407 w409]
          tunnel: w395 -> [_ _]
          tunnel: [w407 w414] -> w393
          tunnel: w397 -> [w404 w408]
          tunnel: [FALSE TRUE] -> w399
          tunnel: [Ass._Loop_Control."Wait" ("Enum") Ass._Loop_Control."SaveReport " ("Enum")] -> w398
          tunnel: [w404 w411] -> w396
          frame 0, Default {
            # "cycyle not ok"
          }
          frame 1 {
            # "Cycle OK"
            n137 = disable-structure shown="Enabled" {
              disable-tunnel: [w429 w440] -> w414
              disable-tunnel: [w427 w438] -> w411
              disable-tunnel: [w426 w442] -> w410
              disable-tunnel: w409 -> [w424 w441]
              disable-tunnel: w408 -> [w415 w439]
              frame Disabled {
                n138 = Unbundle By Name(w415) -> ("Station1 printer IP"=w416:string, "Part PRN path"=w417:path, "Serial_Number"=w418:path)
                n139 = call "Serial_ini.vi"("error in"=w424, "Serial path"=w418, "Enum"=enum16{"Write", "Read"}."Read") -> ("error out"=w425:errorcluster, "Count"=w422:u32)  [unwired: 5 in, 2 out]
                n140 = Increment(x=w422) -> (x+1=w421:u32)
                n141 = Number To Decimal String(number=w421) -> (decimal integer string=w420:string)  [unwired: 1 in]
                n142 = Bundle By Name(cluster=w415, "Current Serial Number"=w420) -> (w419:T4)
                n143 = call "PRN Generation_Station1.vi"("Part PRN QR"=w417, "error in (no error)"=w425, "Cluster"=w419) -> ("QR Code"=w426:string, "PRN to Print"=w428:string, "error out"=w430:errorcluster)  [unwired: 5 in]
                n144 = TCP Open Connection(address=w416, remote port or service name=u16 6101, error in (no error)=w430) -> (connection ID=w433:refnum<k5>, error out=w434:errorcluster)  [unwired: 2 in]
                n145 = TCP Write(connection ID=w433, data in=w428, error in (no error)=w434) -> (connection ID out=w431:refnum<k5>, error out=w436:errorcluster)  [unwired: 1 in, 1 out]
                n146 = call "Stall Data Flow.vim"("value in"=w436, "milliseconds to wait"=u32 1000) -> ("value out"=w432:errorcluster)  [unwired: 1 out]
                n147 = TCP Close Connection(connection ID=w431, error in (no error)=w432) -> (error out=w429:errorcluster)  [unwired: 1 in, 1 out]
                n148 = Bundle By Name(cluster=w419, "Station1_QR"=w426) -> (w427:T4)
              }
              frame Enabled {
                # "Current serial number updates"
                n149 = call "NEW_PRN Generation_Station1.vi"("error in (no error)"=w441, "Cluster in"=w439) -> ("error out"=w440:errorcluster, "cluster out"=w438:T4, "QR CODE"=w442:string)  [unwired: 7 in]
              }
            }
            n150 = local write "QR STATION 1"(w410) -> ()
          }
        }
        n151 = local write "RESULT STATION 1"(w399) -> ()
        n152 = call <vilib>:"Simple Error Handler.vi"("type of dialog (OK msg:1)"=w394, "error in (no error)"=w393) -> ("error out"=w392:errorcluster)  [unwired: 3 in, 4 out]
      }
      frame "SaveReport " {
        w447 = T6 1 items=["no dialog", "OK message", "continue or stop message", "OK message + warnings", "continue/stop + warnings"] ("type of dialog (OK msg:1)")
        # "Save Barcode code AND RESULT in SQL"
        n153 = local read "Para Value"() -> (w443:T1)
        n154 = call "Station1_Data_Log.vi"("error in (no error)"=w453, "Para In"=w443, "Cluster"=w451) -> ("error out"=w452:errorcluster)  [unwired: 8 in]
        n155 = Unbundle By Name(w451) -> ("Serial_Number"=w450:path, "Current Serial Number"=w449:string)
        n156 = Decimal String To Number(string=w449, default (0L)=u32 0 ("default (0 I32)")) -> (number=w444:u32)  [unwired: 1 in, 1 out]
        "SERIAL NO.:- 2" <- w444
        n157 = disable-structure shown="Enabled" {
          disable-tunnel: w452 -> [w461 w464]
          disable-tunnel: w450 -> [w459 _]
          disable-tunnel: [w456 w464] -> w446
          disable-tunnel: w444 -> [w455 _]
          frame Disabled {
            n158 = call "Serial_ini.vi"("error in"=w461, "Serial path"=w459, "Enum"=enum16{"Write", "Read"}."Read") -> ("error out"=w462:errorcluster, "Shift"=w457:string, "Date"=w458:string)  [unwired: 5 in, 1 out]
            n159 = call "Serial_ini.vi"("error in"=w462, "Serial path"=w459, "Date"=w458, "Count"=w455, "Shift"=w457, "Enum"=enum16{"Write", "Read"}."Write") -> ("error out"=w456:errorcluster)  [unwired: 2 in, 3 out]
          }
          frame Enabled {
            # "new modification. no\ngenerate serial number"
          }
        }
        n160 = call <vilib>:"Simple Error Handler.vi"("type of dialog (OK msg:1)"=w447, "error in (no error)"=w446) -> ("error out"=w445:errorcluster)  [unwired: 3 in, 4 out]
      }
      frame "Cycle End" {
      }
      frame "Stop" {
        n161 = local write "CYCLE STATUS STATION 1"("STATION STOP" ("Cycle Status")) -> ()
      }
    }
    n162 = call "TAT_LABVIEW_TO_PLC.vi"("Enum"=enum16{"Read", "Write"}."Write", "error in (no error)"=w83, "Array"=bool[] [TRUE] ("new element/subarray")) -> ()  [unwired: 7 in, 2 out]
    n163 = call "TAT_PLC_Data_read.vi"("Enum"=enum16{"Read", "Write"}."Read") -> ("Array 2"=w85:u16[])  [unwired: 9 in, 1 out]
    n164 = Decimate 1D Array(w85) -> (w84:u16[])  [unwired: 1 out]
    n165 = Index Array(array=w84, index #2=1 ("index")) -> (element #2=w93:u16, element #3=w90:u16, element #4=→"CYCLE TIME:-":u16)  [unwired: 3 in, 1 out]
    n166 = case shown="0, Default" w93 {
      tunnel: [FALSE TRUE] -> w92
      frame 0, Default {
      }
      frame 1 {
      }
    }
    "CYCLE START:-" <- w92
    n167 = call "Parameter_read.vi"("Array"=w84) -> ("Para out"=→"Para Value":T1)  [unwired: 10 in]
    n168 = case shown="0, Default" w90 {
      tunnel: [FALSE TRUE] -> w88
      frame 0, Default {
      }
      frame 1 {
      }
    }
    "CYCLE RESULT:-" <- w88
    n169 = global read "Global 1.vi" "PLC Communication"() -> (→"PLC STATUS:-":bool)
    n170 = Get Date/Time String(want seconds? (F)=TRUE) -> (date string=w110:string, time string=w109:string)  [unwired: 2 in]
    n171 = Concatenate Strings(w110, "\n", w109) -> (→"DATE/TIME":string)
    n172 = Select(t=Ass._Loop_Control."Stop" ("Enum"), s="Stop", f=w98) -> (s? t:f=w99:T5)
    n173 = Wait (ms)(milliseconds to wait=u32 150) -> ()  [unwired: 1 out]
    n174 = Select(t=Ass._Loop_Control."Stop" ("Enum"), s="Stop", f=w96) -> (s? t:f=w113:T5)
  }
  n175 = Merge Errors(w46, w38) -> (w44:errorcluster)
  n176 = Unbundle By Name(w16) -> ("connection reference"=w17:T2)
  n177 = call <vilib>:"Simple Error Handler.vi"("type of dialog (OK msg:1)"=w41, "error in (no error)"=w44) -> ("error out"=w1:errorcluster)  [unwired: 3 in, 4 out]
  "error out" <- w1
  n178 = call <vilib>:"Clear Errors.vi"("error in (no error)"=w1) -> ("error out"=w24:errorcluster)  [unwired: 5 in, 1 out]
  n179 = call <vilib>:"Clear Errors.vi"("error in (no error)"=w1) -> ("error out"=w18:errorcluster)  [unwired: 5 in, 1 out]
  n180 = call "TAT_LABVIEW_TO_PLC.vi"("Enum"=enum16{"Read", "Write"}."Write", "error in (no error)"=w24, "Array"=bool[] [FALSE] ("new element/subarray")) -> ("error out"=w3:errorcluster)  [unwired: 7 in, 1 out]
  n181 = call <vilib>:"DB Tools Close Connection.vi"("error in (no error)"=w18, "connection reference"=w17) -> ("error out"=w2:errorcluster)  [unwired: 5 in]
  n182 = property class="App"() -> ("App.Kind"=w37:T7)  [unwired: 2 in, 2 out]
  n183 = Merge Errors(w3, w1, w2) -> (w4:errorcluster)
  n184 = case shown="\"Run Time System\"" w37 {
    tunnel: w4 -> [_ w474]
    frame "invalid app kind", Default {
    }
    frame "Run Time System" {
      n185 = call <vilib>:"Clear Errors.vi"("error in (no error)"=w474) -> ("error out"=w473:errorcluster)  [unwired: 5 in, 1 out]
      n186 = invoke class="VI" method="FP.Close"(error in=w473) -> ()  [unwired: 2 in, 3 out]
    }
  }
  "CYCLE STATUS STATION 1" <- ""
  "QR STATION 1" <- ""
  "RESULT STATION 1" <- FALSE ("want seconds? (F)")
